vi "liquid_temp_psat.vi"(1 "Liquid Temp [C]":dbl[](array[numeric])) -> (0 "Psat Liquid":dbl[](array[numeric]))   [LabVIEW 2017]
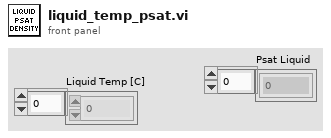
[diagram p1: front panel]
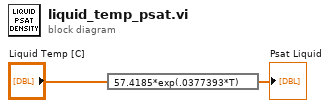
[diagram p0: block diagram]
diagram:
  n1 = expression code="57.4185*exp(.0377393*T)"("Liquid Temp [C]") -> (→"Psat Liquid":dbl[])
